vi "Inital Slope.vi"(10 "H":dbl[](array[numeric]), 11 "B":dbl[](array[numeric])) -> (1 "average slope":dbl, 2 "Downward slope":dbl, 3 "upward slope":dbl)   [LabVIEW 2019]
uses:
  <vilib>/gmath/NI_Gmath.lvlib
  <vilib>/Analysis/NI_AALPro.lvlib
panel:
  out "XY Graph":cluster{"data":dbl[], "data":dbl[]}(graph)
  out "x 1":dbl[](array[numeric])
  out "y1":dbl[](array[numeric])
  out "x2":dbl[](array[numeric])
  out "y2":dbl[](array[numeric])
  out "array size":i32
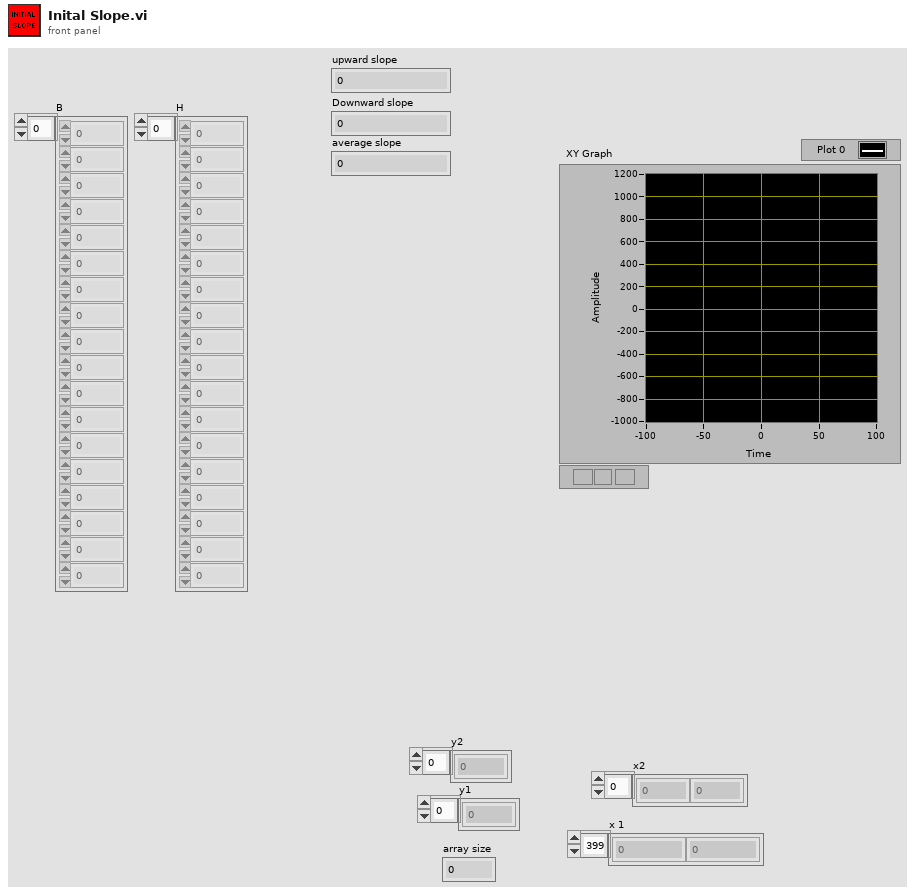
[diagram p1: front panel]
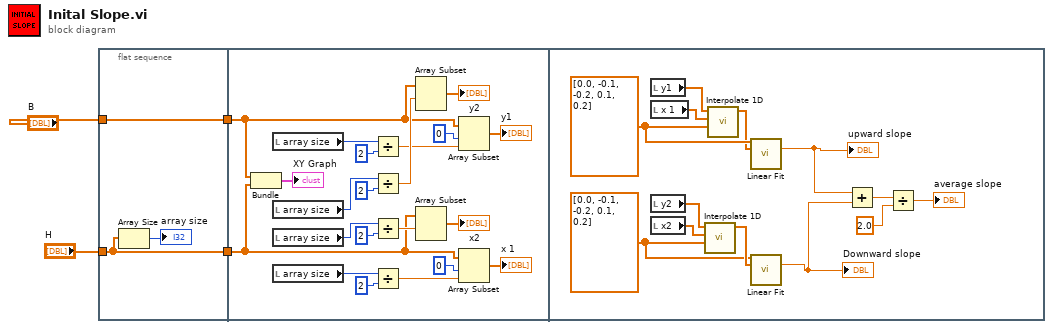
[diagram p0: block diagram]
diagram:
  n1 = flat-sequence {
    tunnel: "H" -> [w5]
    tunnel: "B" -> [w7]
    tunnel: [w7] -> w4
    tunnel: [w5] -> w3
    tunnel: w4 -> [w9]
    tunnel: w3 -> [w8]
    frame #0 {
      n2 = Array Size(array=w5) -> (size(s)=→"array size":i32)
    }
    frame #1 {
      n3 = Bundle("B"=w9, "H"=w8) -> (→"XY Graph":cluster{"B":dbl[], "H":dbl[]})  [unwired: 1 in]
      n4 = local read "array size"() -> (w17:i32)
      n5 = local read "array size"() -> (w25:i32)
      n6 = local read "array size"() -> (w20:i32)
      n7 = local read "array size"() -> (w12:i32)
      n8 = Divide(x=w17, y=2) -> (x/y=w15:dbl)
      n9 = Divide(x=w25, y=2) -> (x/y=w23:dbl)
      n10 = Divide(x=w20, y=2) -> (x/y=w22:dbl)
      n11 = Divide(x=w12, y=2) -> (x/y=w14:dbl)
      n12 = Array Subset(array=w9, index=w23) -> (→"y2":dbl[])  [unwired: 1 in]
      n13 = Array Subset(array=w8, index=w22) -> (→"x2":dbl[])  [unwired: 1 in]
      n14 = Array Subset(array=w9, index=0, length=w15) -> (→"y1":dbl[])
      n15 = Array Subset(array=w8, index=0, length=w14) -> (→"x 1":dbl[])
    }
    frame #2 {
      w34 = dbl[] [0.0, -0.1, -0.2, 0.1, 0.2] ("xi")
      w37 = dbl[] [0.0, -0.1, -0.2, 0.1, 0.2] ("xi")
      n16 = local read "y1"() -> (w38:dbl[])
      n17 = local read "x 1"() -> (w39:dbl[])
      n18 = local read "y2"() -> (w41:dbl[])
      n19 = local read "x2"() -> (w40:dbl[])
      n20 = call <vilib>:"Interpolate 1D.vi"("xi"=w34, "X"=w40, "Y"=w41) -> ("yi"=w35:dbl[])  [unwired: 6 in, 2 out]
      n21 = call <vilib>:"Interpolate 1D.vi"("xi"=w37, "X"=w39, "Y"=w38) -> ("yi"=w36:dbl[])  [unwired: 6 in, 2 out]
      n22 = call <vilib>:"Linear Fit.vi"("Y"=w37, "X"=w36) -> ("slope"=w33:dbl)  [unwired: 9 in, 4 out]
      "upward slope" <- w33
      n23 = call <vilib>:"Linear Fit.vi"("Y"=w34, "X"=w35) -> ("slope"=w32:dbl)  [unwired: 9 in, 4 out]
      "Downward slope" <- w32
      n24 = Add(x=w33, y=w32) -> (x+y=w31:dbl)
      n25 = Divide(x=w31, y=2.0) -> (x/y=→"average slope":dbl)
    }
  }
